vi "Setup Check Scales (SubVI).vi"(6 "[error source] (\" \")":string, 7 "Labels Array":string[](array[string]), 8 "error in (no error)":errorcluster, 9 "[error source] (\" \") 2":string, 10 "Scale Array":tag[](array[tag]), 11 "Channel Array":tag[](array[tag])) -> (0 "error out":errorcluster, 2 "Array of Clusters Out":T1(array[cluster]))   [LabVIEW 2012]
uses:
  <vilib>/Utility/error.llb/DialogType.ctl
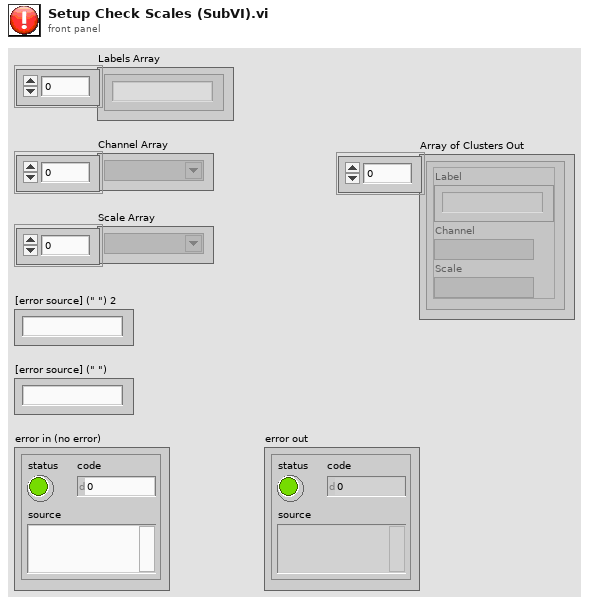
[diagram p1: front panel]
types:
  T1 = cluster{"Label":string, "Channel":tag, "Scale":tag}[]
  T2 = typedef "DialogType.ctl" = u16
  T3 = cluster{"Label":string, "Channel":tag, "Scale":tag}
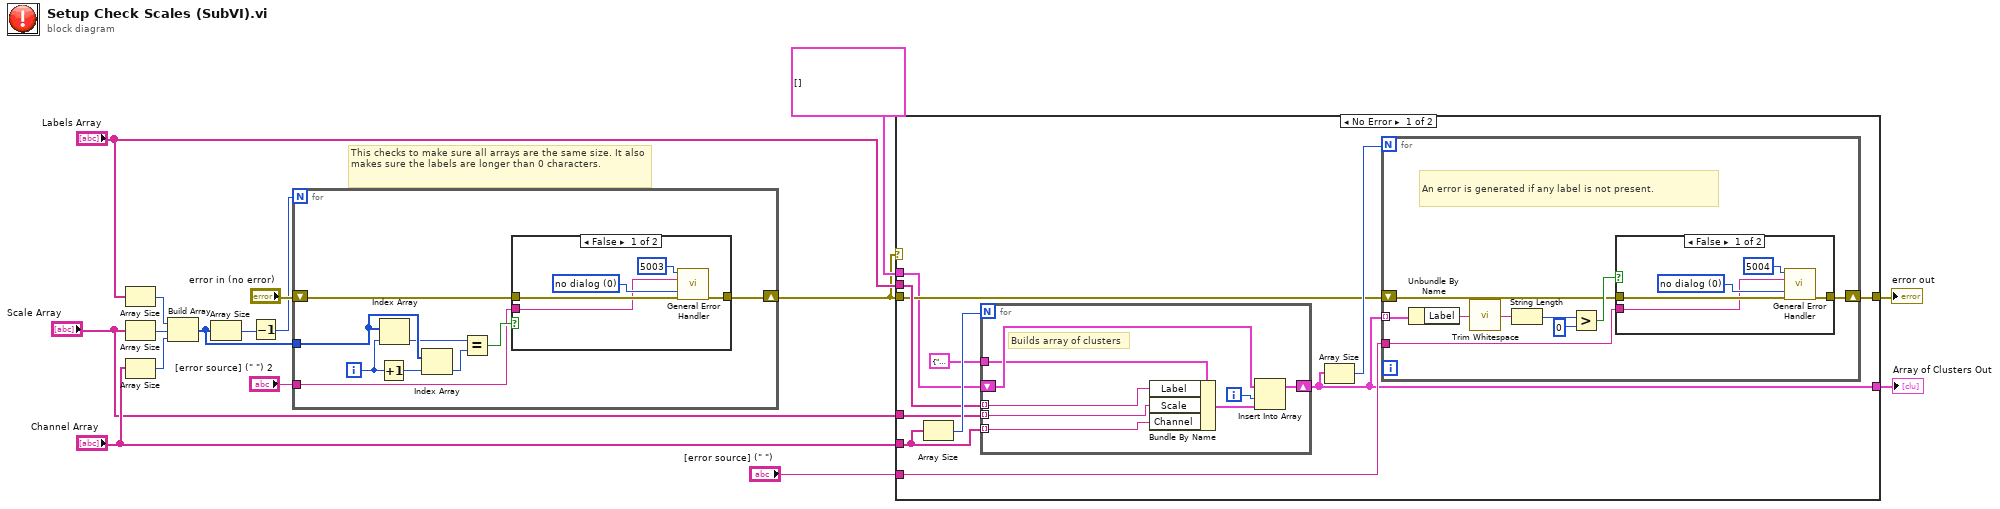
[diagram p0: block diagram]
diagram:
  # "This checks to make sure all arrays are the same size. It also makes sure the labels are longer than 0 characters."
  n1 = Array Size(array="Labels Array") -> (size(s)=w3:i32)
  n2 = Array Size(array="Scale Array") -> (size(s)=w4:i32)
  n3 = Array Size(array="Channel Array") -> (size(s)=w5:i32)
  n4 = Build Array(w3, w4, w5) -> (w9:i32[])
  n5 = Array Size(array=w9) -> (size(s)=w6:i32)
  n6 = Decrement(x=w6) -> (x-1=w7:i32)
  n7 = for {
    N: w7 -> [_]
    tunnel: w9 -> [w25]
    tunnel: "[error source] (\" \") 2" -> [w17]
    shift-right: [w18] -> w11
    shift-left: "error in (no error)" -> [w19]
    i -> [w23]
    n8 = Increment(x=w23) -> (x+1=w24:i32)
    n9 = Index Array(array=w25, index=w23) -> (element=w22:i32)
    n10 = Index Array(array=w25, index=w24) -> (element=w21:i32)
    n11 = Equal?(x=w22, y=w21) -> (x = y?=w20:bool)
    n12 = case shown="False" w20 {
      tunnel: w19 -> [w30 w31]
      tunnel: [w29 w31] -> w18
      tunnel: w17 -> [w26 _]
      frame False {
        w28 = T2 0 items=["no dialog", "OK message", "continue or stop message", "OK message + warnings", "continue/stop + warnings"] ("type of dialog (OK msg:1)")
        n13 = call <vilib>:"General Error Handler.vi"("[error code] (0)"=5003, "[error source] (\" \")"=w26, "type of dialog (OK msg:1)"=w28, "error in (no error)"=w30) -> ("error out"=w29:errorcluster)  [unwired: 7 in, 4 out]
      }
      frame True {
      }
    }
  }
  n14 = case shown="No Error" w11 {
    tunnel: "Labels Array" -> [w40 _]
    tunnel: "Scale Array" -> [w32 _]
    tunnel: "Channel Array" -> [w41 _]
    tunnel: [w36 w67] -> w13
    tunnel: w11 -> [w37 w67]
    tunnel: "[error source] (\" \")" -> [w38 _]
    tunnel: T1 [] -> [w35 w66]
    tunnel: [w34 w66] -> w1
    frame No Error {
      n15 = Array Size(array=w41) -> (size(s)=w42:i32)
      n16 = for {
        N: w42 -> [_]
        tunnel: w41 -> [w65] mode=indexing
        tunnel: w40 -> [w64] mode=indexing
        shift-right: [w63] -> w34
        shift-left: w35 -> [w62]
        tunnel: T3 {"Label"="", "Channel"="", "Scale"=""} -> [w60]
        tunnel: w32 -> [w58] mode=indexing
        i -> [w61]
        # "Builds array of clusters"
        n17 = Bundle By Name(cluster=w60, "Label"=w64, "Scale"=w58, "Channel"=w65) -> (w59:T3)
        n18 = Insert Into Array(array=w62, index=w61, new element=w59) -> (w63:T1)
      }
      n19 = Array Size(array=w34) -> (size(s)=w39:i32)
      n20 = for {
        N: w39 -> [_]
        tunnel: w34 -> [w51] mode=indexing
        shift-right: [w44] -> w36
        shift-left: w37 -> [w45]
        tunnel: w38 -> [w43]
        # "An error is generated if any label is not present."
        n21 = Unbundle By Name(w51) -> ("Label"=w50:string)
        n22 = call <vilib>:"Trim Whitespace.vi"("string"=w50) -> ("trimmed string"=w49:string)  [unwired: 1 in]
        n23 = String Length(string=w49) -> (length=w48:i32)
        n24 = Greater?(x=w48, y=0) -> (0:w46:bool)
        n25 = case shown="False" w46 {
          tunnel: w45 -> [w54 w57]
          tunnel: [w53 w57] -> w44
          tunnel: w43 -> [w52 _]
          frame False {
            w55 = T2 0 items=["no dialog", "OK message", "continue or stop message", "OK message + warnings", "continue/stop + warnings"] ("type of dialog (OK msg:1)")
            n26 = call <vilib>:"General Error Handler.vi"("[error code] (0)"=5004, "[error source] (\" \")"=w52, "type of dialog (OK msg:1)"=w55, "error in (no error)"=w54) -> ("error out"=w53:errorcluster)  [unwired: 7 in, 4 out]
          }
          frame True {
          }
        }
      }
    }
    frame Error {
    }
  }
  "error out" <- w13
  "Array of Clusters Out" <- w1
